vi "dfd_Modulus from Ratio.vi"(0 "u":dbl=1.0 format="%.2f") -> (1 "fk(u)":dbl format="%.4f", 2 "convergence":bool=TRUE)   [LabVIEW 2017, in "NI_DigFilter_Design.lvlib"]
uses:
  <vilib>/addons/Digital Filter Design/NI_DigFilter_Design.lvlib
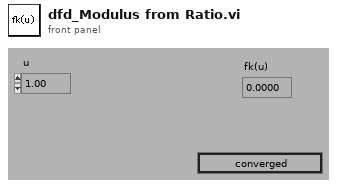
[diagram p1: front panel]
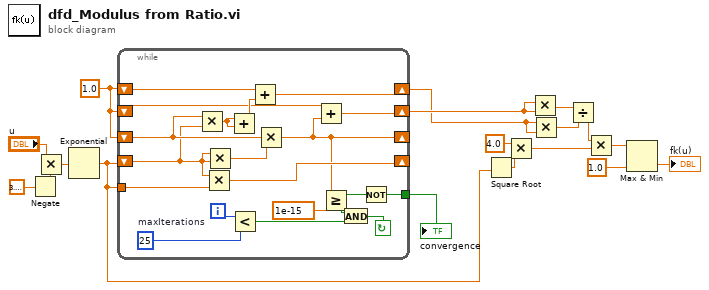
[diagram p0: block diagram]
diagram:
  w17 = 1.0
  n1 = Negate(x=3.141592653589793) -> (-x=w15:dbl)
  n2 = Multiply(x="u", y=w15) -> (x*y=w13:dbl)
  n3 = Exponential(1:w13) -> (0:w11:dbl)
  n4 = while {
    tunnel: w11 -> [w27]
    shift-left: w11 -> [w28]
    shift-right: [w26] -> _
    shift-left: w17 -> [w20]
    shift-right: [w19] -> w9
    tunnel: [w32] -> w18
    shift-left: w17 -> [w29]
    shift-right: [w21] -> _
    shift-left: w17 -> [w23]
    shift-right: [w22] -> w8
    i -> [w37]
    stop <- w33 continue-if-true
    w31 = 25  # maxIterations
    n5 = Multiply(x=w29, y=w28) -> (x*y=w25:dbl)
    n6 = Multiply(x=w28, y=w27) -> (x*y=w26:dbl)
    n7 = Multiply(x=w28, y=w28) -> (x*y=w30:dbl)
    n8 = Add(x=w25, y=w25) -> (x+y=w24:dbl)
    n9 = Less?(x=w37, y=w31) -> (x < y?=w34:bool)
    n10 = Add(x=w23, y=w24) -> (x+y=w22:dbl)
    n11 = Multiply(x=w29, y=w30) -> (x*y=w21:dbl)
    n12 = Add(x=w20, y=w21) -> (x+y=w19:dbl)
    n13 = Greater Or Equal?(x=w21, y=1e-15) -> (x >= y?=w35:bool)
    n14 = And(x=w35, y=w34) -> (x .and. y?=w33:bool)
    n15 = Not(x=w35) -> (.not. x?=w32:bool)
  }
  "convergence" <- w18
  n16 = Square Root(x=w11) -> (sqrt(x)=w10:dbl)
  n17 = Multiply(x=4.0, y=w10) -> (x*y=w4:dbl)
  n18 = Multiply(x=w9, y=w9) -> (x*y=w6:dbl)
  n19 = Multiply(x=w8, y=w8) -> (x*y=w7:dbl)
  n20 = Divide(x=w6, y=w7) -> (x/y=w5:dbl)
  n21 = Multiply(x=w5, y=w4) -> (x*y=w3:dbl)
  n22 = Max & Min(x=w3, y=1.0) -> (min(x,y)=→"fk(u)":dbl)  [unwired: 1 out]
